vi "Merge Overlapping Regions.vi"(10 "Regions width":dbl, 11 "Region centers":dbl[](array[numeric])) -> (2 "Region widths out":dbl[](array[numeric]), 3 "Region centers out":dbl[](array[numeric]))   [LabVIEW 2016]
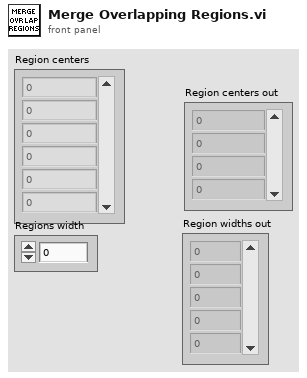
[diagram p1: front panel]
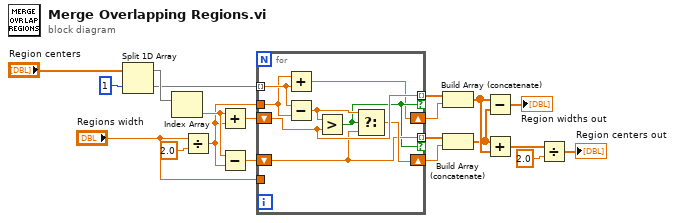
[diagram p0: block diagram]
diagram:
  n1 = Split 1D Array(array="Region centers", index=1) -> (first subarray=w13:dbl[], second subarray=w12:dbl[])
  n2 = Index Array(array=w13) -> (element=w8:dbl)  [unwired: 1 in]
  n3 = Divide(x="Regions width", y=2.0) -> (x/y=w7:dbl)
  n4 = Add(x=w8, y=w7) -> (x+y=w11:dbl)
  n5 = Subtract(x=w8, y=w7) -> (x-y=w9:dbl)
  n6 = for {
    shift-right: [w22] -> w4
    shift-left: w11 -> [w28]
    tunnel: w12 -> [w24] mode=indexing
    tunnel: "Regions width" -> [_]
    tunnel: [w28] -> w6 mode=indexing if=w23
    shift-right: [w27] -> w3
    shift-left: w9 -> [w25]
    tunnel: [w25] -> w1 mode=indexing if=w23
    tunnel: w7 -> [w21]
    n7 = Add(x=w21, y=w24) -> (x+y=w22:dbl)
    n8 = Subtract(x=w24, y=w21) -> (x-y=w26:dbl)
    n9 = Greater?(x=w26, y=w28) -> (0:w23:bool)
    n10 = Select(t=w26, s=w23, f=w25) -> (s? t:f=w27:dbl)
  }
  n11 = Build Array (concatenate)(w6, w4) -> (w5:dbl[])
  n12 = Build Array (concatenate)(w1, w3) -> (w2:dbl[])
  n13 = Subtract(x=w5, y=w2) -> (x-y=→"Region widths out":dbl[])
  n14 = Add(x=w2, y=w5) -> (x+y=w20:dbl[])
  n15 = Divide(x=w20, y=2.0) -> (x/y=→"Region centers out":dbl[])
